vi "User Interface.vi"() -> ()   [LabVIEW 2009]
uses:
  UDP Lib/UDP Network Location.ctl
  Motor Command.ctl
  Debug Shared/Debug Data Packet.ctl
  TypeDefs/State Machine/Main State.ctl
  cRIO/Functional Global Variables/Status Indicators.ctl
  TypeDefs/Sensor TypeDefs/GPS Data.ctl
  TypeDefs/Sensor TypeDefs/SICK Array.ctl
  TypeDefs/Queue TypeDefs/Motor Instruction.ctl
  TypeDefs/Queue TypeDefs/Motor State.ctl
  Control Message.ctl
  UI States.ctl
  <vilib>/Utility/inputDevices.llb/joystickAcquire.vi
  <vilib>/Utility/inputDevices.llb/closeJoystick.vi
panel:
  out "EVS HB":bool
  out "Batt Voltage":dbl
  out "Bearing Graph":cluster{dbl[], dbl[]}[](graph)
  out "Sector Graph":cluster{dbl[], dbl[]}[](graph)
  in  "Parameters":T1={"Turn deadzone"=8000, "Turn scaling factor"=1500, "Speed scaling factor "=400, "Speed deadzone "=8000}
  out "All stop":bool=TRUE
  out "Speed":i32(slide) min=-127 max=127 step=1 scale=-127.0..127.0
  out "Turn":i32(slide) min=-127 max=127 step=1 scale=-127.0..127.0
  in  "Pause Motors":bool
  out "SICK Data":T2(graph)
  out "Loop Period":u32=1
  out "status":bool
  in  "Debug Request":bool
  in  "Debug Location":T3={"IP Address"="192.168.1.2", "Port"=50004}
  out "Debug Data":T4={"Main State out"=enum."Initialize Sensors", "HB out"=FALSE, "Status Indicators out"={"GPS Init Complete"=FALSE, "SICK Init Complete"=FALSE, "Compass Init Complete"=FALSE, "Camera Init Complete"=FALSE, "Sensors Init Complete"=FALSE, "Motors Init Complete"=FALSE, "MC Heartbeat"=FALSE, "Motors On?"=FALSE, "Encoders Zeroed?"=FALSE, "JAUS Go"=FALSE}, "RC/!Run out"=FALSE, "AUT/!NAV"=FALSE, "Compass Data"=0.0, "GPS Data"={"Latitude"=0.0, "Longitude"=0.0}, "SICK Data"=[], "Target Bearing"=0.0, "Target Sector"=0, "Calculated sector"=0, "RC Command"={"Speed"=0, "Turn"=0}, "Motor Loop Instruction"={"Motor State"=enum."Stop", "Motor Command"={"Speed"=0, "Turn"=0}}, "Waypoints reached"=0, "Battery Voltage"=0.0, "Local Pose"={"X Coordinate"=0.0, "Y Coordinate"=0.0}, "EVS HB"=FALSE} {"GPS Data"."Longitude" format="%#_14g"; "GPS Data"."Latitude" format="%#_14g"}
  in  "Cluster":T4={"Main State out"=enum."Initialize Sensors", "HB out"=FALSE, "Status Indicators out"={"GPS Init Complete"=FALSE, "SICK Init Complete"=FALSE, "Compass Init Complete"=FALSE, "Camera Init Complete"=FALSE, "Sensors Init Complete"=FALSE, "Motors Init Complete"=FALSE, "MC Heartbeat"=FALSE, "Motors On?"=FALSE, "Encoders Zeroed?"=FALSE, "JAUS Go"=FALSE}, "RC/!Run out"=FALSE, "AUT/!NAV"=FALSE, "Compass Data"=0.0, "GPS Data"={"Latitude"=0.0, "Longitude"=0.0}, "SICK Data"=[], "Target Bearing"=0.0, "Target Sector"=0, "Calculated sector"=0, "RC Command"={"Speed"=0, "Turn"=0}, "Motor Loop Instruction"={"Motor State"=enum."Stop", "Motor Command"={"Speed"=0, "Turn"=0}}, "Waypoints reached"=0, "Battery Voltage"=0.0, "Local Pose"={"X Coordinate"=0.0, "Y Coordinate"=0.0}, "EVS HB"=FALSE} {"GPS Data"."Longitude" format="%#_14g"; "GPS Data"."Latitude" format="%#_14g"}
  in  "Remote Control?":bool
  in  "Read Debug?":bool
  in  "stop":bool
  out "Motor Command":T8
  in  "cRIO Network Location":T3={"IP Address"="192.168.1.2", "Port"=50001}
  # "UI Control"
  # "Xbox RC"
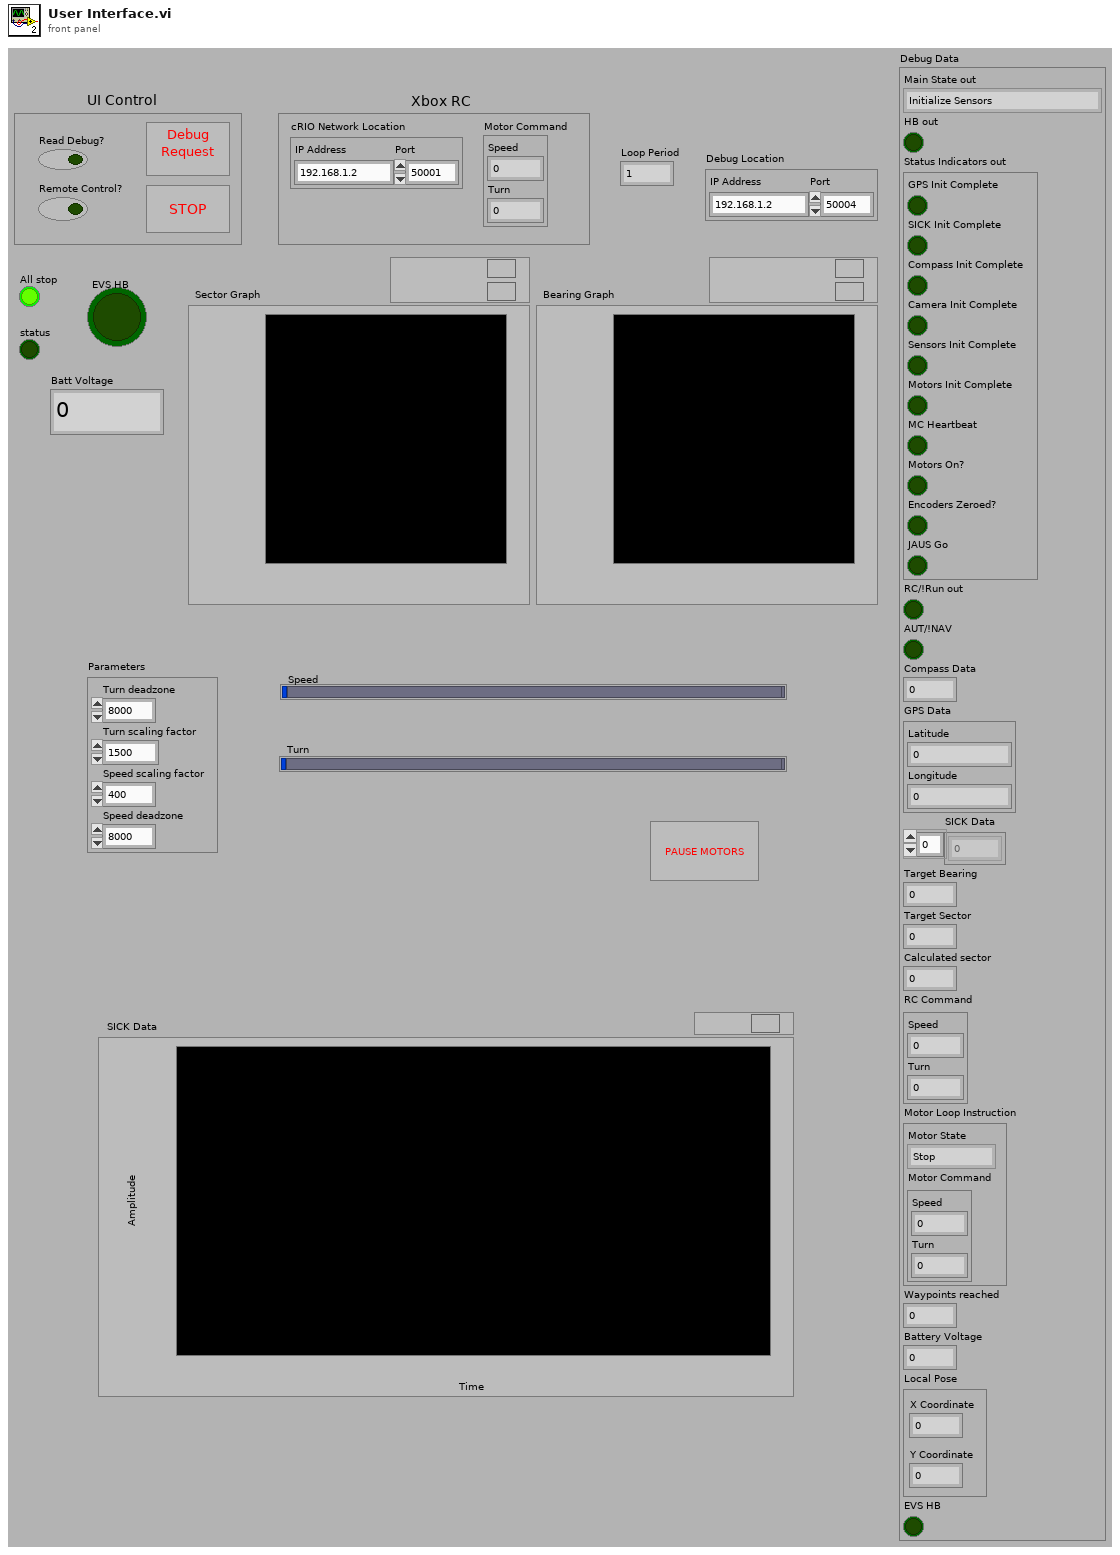
[diagram p1: front panel]
types:
  T1 = cluster{"Turn deadzone":i32, "Turn scaling factor":i32, "Speed scaling factor ":i32, "Speed deadzone ":i32}
  T2 = typedef "SICK Array.ctl" = u16[]
  T3 = typedef "UDP Network Location.ctl" = cluster{"IP Address":string, "Port":u16}
  T4 = typedef "Debug Data Packet.ctl" = cluster{"Main State out":T5, "HB out":bool, "Status Indicators out":T6, "RC/!Run out":bool, "AUT/!NAV":bool, "Compass Data":dbl, "GPS Data":T7, "SICK Data":T2, "Target Bearing":dbl, "Target Sector":i16, "Calculated sector":i16, "RC Command":T8, "Motor Loop Instruction":T9, "Waypoints reached":i8, "Battery Voltage":dbl, "Local Pose":cluster{"X Coordinate":dbl, "Y Coordinate":dbl}, "EVS HB":bool}
  T5 = typedef "Main State.ctl" = enum16{"Startup", "Wait for Init", "Initialize Sensors", "Wait for Saftey Disable", "Check Saftey", "Wait for GO", "Run", "Remote Control", "Stop"}
  T6 = typedef "Status Indicators.ctl" = cluster{"GPS Init Complete":bool, "SICK Init Complete":bool, "Compass Init Complete":bool, "Camera Init Complete":bool, "Sensors Init Complete":bool, "Motors Init Complete":bool, "MC Heartbeat":bool, "Motors On?":bool, "Encoders Zeroed?":bool, "JAUS Go":bool}
  T7 = typedef "GPS Data.ctl" = cluster{"Latitude":dbl, "Longitude":dbl}
  T8 = typedef "Motor Command.ctl" = cluster{"Speed":i16, "Turn":i16}
  T9 = typedef "Motor Instruction.ctl" = cluster{"Motor State":T10, "Motor Command":T8}
  T10 = typedef "Motor State.ctl" = enum16{"Wait", "Initialize", "Check FET", "Run", "Stop"}
  T11 = typedef "Control Message.ctl" = cluster{"Motor Command":T8, "Time Stamp":timestamp, "Remote  Control/!Autonomous":bool, "Send Debug Data?":bool}
  T12 = typedef "UI States.ctl" = enum16{"Send Motor Command", "Read Debug Data", "Do Nothing", "Request Debug Control"}
  T13 = typedef "UDP Base.ctl" = cluster{"UDP Session":refnum<k16>, "UDP Socket Params":T14}
  T14 = typedef "UDP Socket Params.ctl" = cluster{"Local Port":u16, "Read Timeout":i32, "Write Timeout":i32}
  T15 = cluster{"X axis":i32, "Y axis":i32, "Z axis":i32, "X axis rotation":i32, "Y axis rotation":i32, "Z axis rotation":i32, "U axis":i32, "V axis":i32}
  T16 = cluster{"button 1":bool, "button 2":bool, "button 3":bool, "button 4":bool, "button 5":bool, "button 6":bool, "button 7":bool, "button 8":bool, "button 9":bool, "button 10":bool, "button 11":bool, "button 12":bool, "button 13":bool, "button 14":bool, "button 15":bool, "button 16":bool, "button 17":bool, "button 18":bool, "button 19":bool, "button 20":bool, "button 21":bool, "button 22":bool, "button 23":bool, "button 24":bool, "button 25":bool, "button 26":bool, "button 27":bool, "button 28":bool, "button 29":bool, "button 30":bool, "button 31":bool, "button 32":bool}
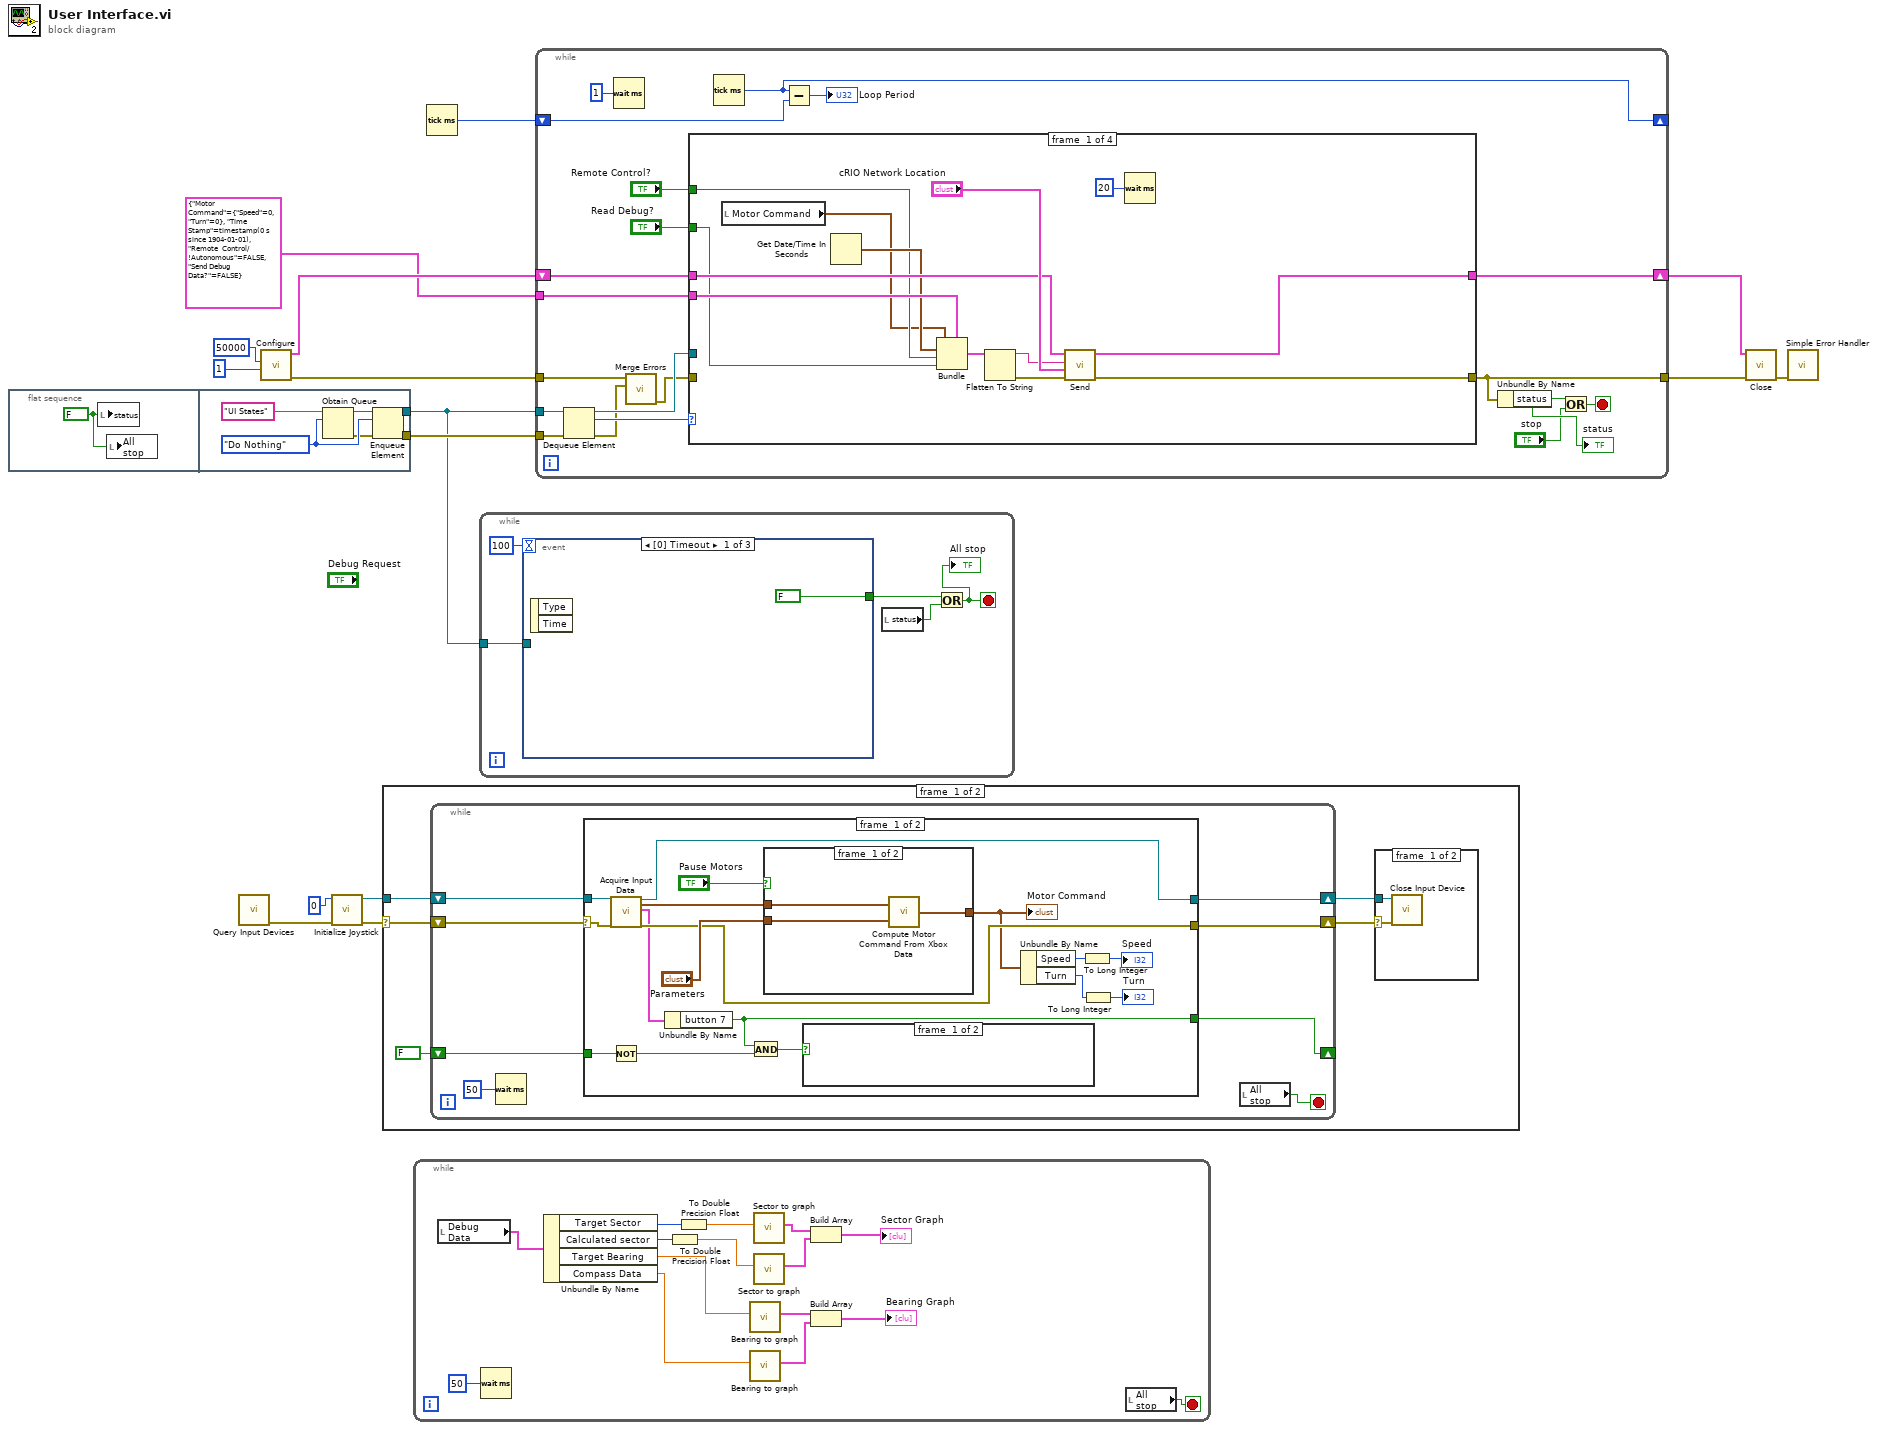
[diagram p0: block diagram]
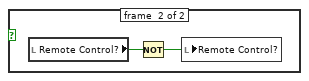
[diagram p3: hidden frame]
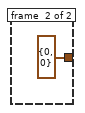
[diagram p4: hidden frame]
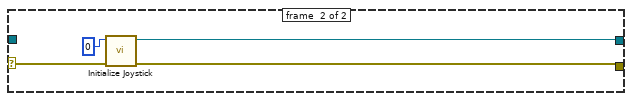
[diagram p5: hidden frame]
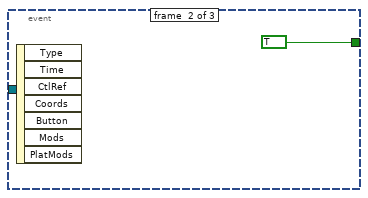
[diagram p7: hidden frame]
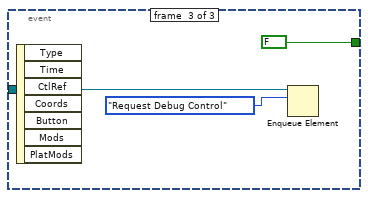
[diagram p8: hidden frame]
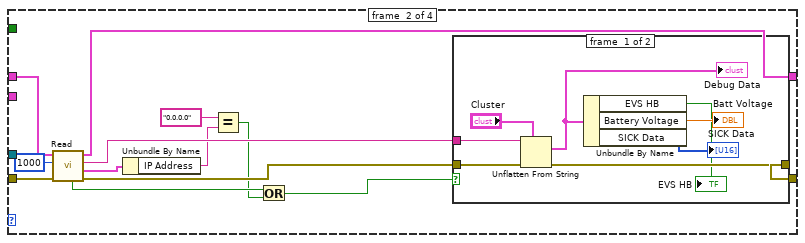
[diagram p9: hidden frame]
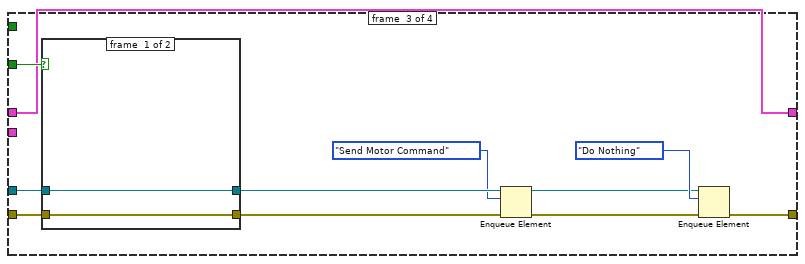
[diagram p11: hidden frame]
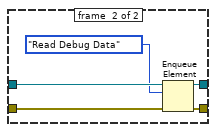
[diagram p12: hidden frame]
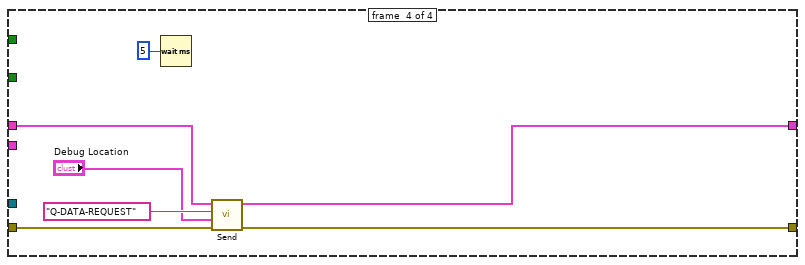
[diagram p13: hidden frame]
diagram:
  n1 = flat-sequence {
    tunnel: [w18] -> w8
    tunnel: [w17] -> w7
    frame #0 {
      w16 = FALSE ("status")
      n2 = local write "status"(w16) -> ()
      n3 = local write "All stop"(w16) -> ()
    }
    frame #1 {
      w21 = UI_States."Do Nothing" ("UI States")
      n4 = Obtain Queue(name (unnamed)="UI States", element data type=w21) -> (queue out=w20:refnum<queue>, error out=w19:errorcluster)  [unwired: 3 in, 1 out]
      n5 = Enqueue Element(queue=w20, element=w21, error in (no error)=w19) -> (queue out=w17:refnum<queue>, error out=w18:errorcluster)  [unwired: 1 in, 1 out]
    }
  }
  n6 = call <vilib>:"Query Input Devices.vi"() -> ("error out"=w5:errorcluster)  [unwired: 1 in, 10 out]
  n7 = call "Configure.vi"("Read Timeout"=1, "Local Port"=u16 50000) -> ("error out"=w4:errorcluster, "UDP Base out"=w13:T13)  [unwired: 8 in]
  n8 = call <vilib>:"Initialize Joystick.vi"("error in (no error)"=w5, "device index"=0) -> ("error out"=w1:errorcluster, "device ID"=w2:refnum<k1>)  [unwired: 8 out]
  n9 = case shown="No Error" w1 {
    selector: w1 -> [w26 _]
    tunnel: w2 -> [w27 _]
    frame #0 {
      n10 = while {
        shift-right: [w33] -> w25
        shift-left: w27 -> [w36]
        shift-right: [w34] -> w24
        shift-left: w26 -> [w32]
        shift-right: [w30] -> _
        shift-left: FALSE ("button 7") -> [w31]
        stop <- w35 stop-if-true
        n11 = Wait (ms)(milliseconds to wait=u32 50) -> ()  [unwired: 1 out]
        n12 = case shown="No Error" w32 {
          selector: w32 -> [w43 w63]
          tunnel: w36 -> [w52 _]
          tunnel: [w51 w61] -> w34
          tunnel: [w50 w62] -> w33
          tunnel: w31 -> [w41 _]
          tunnel: [w38 _] -> w30
          frame #0 {
            n13 = call-poly <vilib>:"Acquire Input Data.vi"("device ID"=w52, "error in (no error)"=w43) -> ("device ID"=w50:refnum<k1>, "axis info"=w53:T15, "button info"=w42:T16, "error out"=w51:errorcluster)  [unwired: 14 out]
            n14 = Not(x=w41) -> (.not. x?=w40:bool)
            n15 = Unbundle By Name(w42) -> ("button 7"=w38:bool)
            n16 = And(x=w38, y=w40) -> (x .and. y?=w39:bool)
            n17 = case shown="False" "Pause Motors" {
              tunnel: "Parameters" -> [w59 _]
              tunnel: w53 -> [w58 _]
              tunnel: [w57 T8 {"Speed"=0, "Turn"=0} ("Motor Command")] -> w48
              frame #0 {
                n18 = call "Compute Motor Command From Xbox Data.vi"("Parameters"=w59, "Xbox Controller Axis Info"=w58) -> ("Motor Command"=w57:T8)
              }
              frame #1 {
              }
            }
            "Motor Command" <- w48
            n19 = case shown="True" w39 {
              frame #0 {
              }
              frame #1 {
                n20 = local read "Remote Control?"() -> (w56:bool)
                n21 = Not(x=w56) -> (.not. x?=w55:bool)
                n22 = local write "Remote Control?"(w55) -> ()
              }
            }
            n23 = Unbundle By Name(w48) -> ("Speed"=w47:i16, "Turn"=w46:i16)
            n24 = To Long Integer(number=w47) -> (32bit integer=→"Speed":i32)
            n25 = To Long Integer(number=w46) -> (32bit integer=→"Turn":i32)
          }
          frame #1 {
            n26 = call <vilib>:"Initialize Joystick.vi"("error in (no error)"=w63, "device index"=0) -> ("error out"=w61:errorcluster, "device ID"=w62:refnum<k1>)  [unwired: 8 out]
          }
        }
        n27 = local read "All stop"() -> (w35:bool)
      }
      n28 = case shown="No Error" w24 {
        selector: w24 -> [w28 _]
        tunnel: w25 -> [w29 _]
        frame #0 {
          n29 = call-poly <vilib>:"Close Input Device.vi"("error in (no error)"=w28, "device ID"=w29) -> ()  [unwired: 9 out]
        }
        frame #1 {
        }
      }
    }
    frame #1 {
    }
  }
  n30 = while {
    stop <- w72 stop-if-true
    n31 = local read "Debug Data"() -> (w78:T4)
    n32 = Wait (ms)(milliseconds to wait=u32 50) -> ()  [unwired: 1 out]
    n33 = Unbundle By Name(w78) -> ("Target Sector"=w77:i16, "Calculated sector"=w76:i16, "Target Bearing"=w65:dbl, "Compass Data"=w71:dbl)
    n34 = To Double Precision Float(number=w76) -> (double precision float=w69:dbl)
    n35 = To Double Precision Float(number=w77) -> (double precision float=w70:dbl)
    n36 = call "Bearing to graph.vi"("Bearing"=w65) -> ("XY Graph"=w68:cluster{dbl[], dbl[]})  [unwired: 10 in]
    n37 = call "Bearing to graph.vi"("Bearing"=w71) -> ("XY Graph"=w67:cluster{dbl[], dbl[]})  [unwired: 10 in]
    n38 = call "Sector to graph.vi"("Sector"=w70) -> ("XY Graph"=w75:cluster{dbl[], dbl[]})  [unwired: 10 in]
    n39 = call "Sector to graph.vi"("Sector"=w69) -> ("XY Graph"=w74:cluster{dbl[], dbl[]})  [unwired: 10 in]
    n40 = Build Array(w75, w74) -> (→"Sector Graph":cluster{dbl[], dbl[]}[])
    n41 = Build Array(w68, w67) -> (→"Bearing Graph":cluster{dbl[], dbl[]}[])
    n42 = local read "All stop"() -> (w72:bool)
  }
  n43 = Tick Count (ms)() -> (millisecond timer value=w6:u32)
  n44 = while {
    tunnel: w7 -> [w82]
    stop <- w81 stop-if-true
    n45 = event shown="[0] Timeout" {
      selector: _ -> [_ _ _]
      dyn-events: _ -> [_ _ _]
      timeout: 100 -> [_ _ _]
      tunnel: [FALSE TRUE FALSE] -> w83
      tunnel: w82 -> [_ _ w89]
      event #0 {
        n46 = event-data() -> ()  [unwired: 1 in, 2 out]
      }
      event #1 {
        n47 = event-data() -> ()  [unwired: 1 in, 7 out]
      }
      event #2 {
        n48 = event-data() -> ()  [unwired: 1 in, 7 out]
        n49 = Enqueue Element(queue=w89, element=UI_States."Request Debug Control") -> ()  [unwired: 2 in, 3 out]
      }
    }
    n50 = local read "status"() -> (w80:bool)
    n51 = Or(x=w83, y=w80) -> (x .or. y?=w81:bool)
    "All stop" <- w81
  }
  n52 = while {
    tunnel: w4 -> [w100]
    shift-right: [w108] -> w11
    shift-left: w13 -> [w109]
    tunnel: [w96] -> w3
    tunnel: T11 {"Motor Command"={"Speed"=0, "Turn"=0}, "Time Stamp"=timestamp(0 s since 1904-01-01), "Remote  Control/!Autonomous"=FALSE, "Send Debug Data?"=FALSE} ("Control Cluster") -> [w107]
    tunnel: w7 -> [w104]
    tunnel: w8 -> [w103]
    shift-right: [w91] -> _
    shift-left: w6 -> [w92]
    stop <- w93 stop-if-true
    n53 = Dequeue Element(queue=w104, error in (no error)=w103) -> (queue out=w101:refnum<queue>, element=w102:T12, error out=w99:errorcluster)  [unwired: 1 in, 1 out]
    n54 = Wait (ms)(milliseconds to wait=u32 1 ("millisecond multiple")) -> ()  [unwired: 1 out]
    n55 = call <vilib>:"Merge Errors.vi"("error in 2 (no error)"=w99, "error in 1 (no error)"=w100) -> ("error out"=w98:errorcluster)  [unwired: 5 in]
    n56 = case shown="\"Read Debug Data\"" w102 {
      tunnel: w98 -> [_ w132 w153 w167]
      tunnel: w109 -> [w121 w135 w147 w168]
      tunnel: [w117 w126 w147 w164] -> w108
      tunnel: [w116 w130 w149 w165] -> w96
      tunnel: w107 -> [w115 _ _ _]
      tunnel: "Read Debug?" -> [w113 _ w155 _]
      tunnel: w101 -> [_ _ w154 _]
      tunnel: "Remote Control?" -> [w112 _ _ _]
      frame #0 {
        n57 = local read "Motor Command"() -> (w111:T8)
        n58 = Get Date/Time In Seconds() -> (seconds since 1Jan1904=w114:timestamp)
        n59 = Bundle(cluster=w115, "Motor Command"=w111, "Time Stamp"=w114, "Remote  Control/!Autonomous"=w112, "Send Debug Data?"=w113) -> (w120:T11)
        n60 = Flatten To String(anything=w120) -> (data string=w118:string, error out=w119:errorcluster)  [unwired: 3 in, 1 out]
        n61 = call "Send.vi"("error in (no error)"=w119, "Destination Location"="cRIO Network Location", "Send Data"=w118, "UDP Base in"=w121) -> ("error out"=w116:errorcluster, "UDP Base out"=w117:T13)  [unwired: 5 in, 1 out]
        n62 = Wait (ms)(milliseconds to wait=u32 20 ("millisecond multiple")) -> ()  [unwired: 1 out]
      }
      frame #1 {
        n63 = call "Read.vi"("error in (no error)"=w132, "max size (548)"=1000, "UDP Base in"=w135) -> ("error out"=w131:errorcluster, "Network Location"=w129:T3, "Receive Data"=w133:string, "UDP Base out"=w126:T13, "Timeout"=w134:bool)  [unwired: 3 in, 1 out]
        n64 = Unbundle By Name(w129) -> ("IP Address"=w127:string)
        n65 = Equal?(x="0.0.0.0", y=w127) -> (x = y?=w125:bool)
        n66 = Or(x=w134, y=w125) -> (x .or. y?=w128:bool)
        n67 = case shown="False" w128 {
          tunnel: w133 -> [w143 _]
          tunnel: w131 -> [w142 w144]
          tunnel: [w141 w144] -> w130
          frame #0 {
            n68 = Unflatten From String(type="Cluster", binary string=w143, error in (no error)=w142) -> (value=w139:T4, error out=w141:errorcluster)  [unwired: 2 in, 1 out]
            "Debug Data" <- w139
            n69 = Unbundle By Name(w139) -> ("EVS HB"=→"EVS HB":bool, "Battery Voltage"=→"Batt Voltage":dbl, "SICK Data"=→"SICK Data":T2)
          }
          frame #1 {
          }
        }
      }
      frame #2 {
        n70 = case shown="True" w155 {
          tunnel: w154 -> [w156 w162]
          tunnel: w153 -> [w157 w161]
          tunnel: [w157 w160] -> w151
          tunnel: [w156 w158] -> w152
          frame #0 {
          }
          frame #1 {
            n71 = Enqueue Element(queue=w162, element=UI_States."Read Debug Data", error in (no error)=w161) -> (queue out=w158:refnum<queue>, error out=w160:errorcluster)  [unwired: 1 in, 1 out]
          }
        }
        n72 = Enqueue Element(queue=w152, element=UI_States."Send Motor Command", error in (no error)=w151) -> (queue out=w148:refnum<queue>, error out=w146:errorcluster)  [unwired: 1 in, 1 out]
        n73 = Enqueue Element(queue=w148, element=UI_States."Do Nothing", error in (no error)=w146) -> (error out=w149:errorcluster)  [unwired: 1 in, 2 out]
      }
      frame #3 {
        n74 = Wait (ms)(milliseconds to wait=u32 5 ("millisecond multiple")) -> ()  [unwired: 1 out]
        n75 = call "Send.vi"("error in (no error)"=w167, "Destination Location"="Debug Location", "Send Data"="Q-DATA-REQUEST", "UDP Base in"=w168) -> ("error out"=w165:errorcluster, "UDP Base out"=w164:T13)  [unwired: 5 in, 1 out]
      }
    }
    n76 = Tick Count (ms)() -> (millisecond timer value=w91:u32)
    n77 = Subtract(x=w91, y=w92) -> (x-y=→"Loop Period":u32)
    n78 = Unbundle By Name(w96) -> ("status"=w95:bool)
    "status" <- w95
    n79 = Or(x=w95, y="stop") -> (x .or. y?=w93:bool)
  }
  n80 = call "Close.vi"("error in (no error)"=w3, "Cluster of class private data"=w11) -> ("error out"=w10:errorcluster)  [unwired: 9 in]
  n81 = call <vilib>:"Simple Error Handler.vi"("error in (no error)"=w10) -> ()  [unwired: 1 in, 8 out]
